vi "Runtime_Check.vi"(1 "Machine Settings":cluster{"Max Value":dbl, "Min Value":dbl}, 5 "Initial Timestamp":timestamp, 6 "error in (no error)":errorcluster, 7 "Tolerance":dbl, 8 "setpoint profile":cluster{"time (s)":dbl, "setpoint":dbl}[](array[cluster]), 9 "Process_REF":string) -> (0 "error out":errorcluster, 3 "Path Out":path)   [LabVIEW 2018]
panel:
  in  "stop":bool
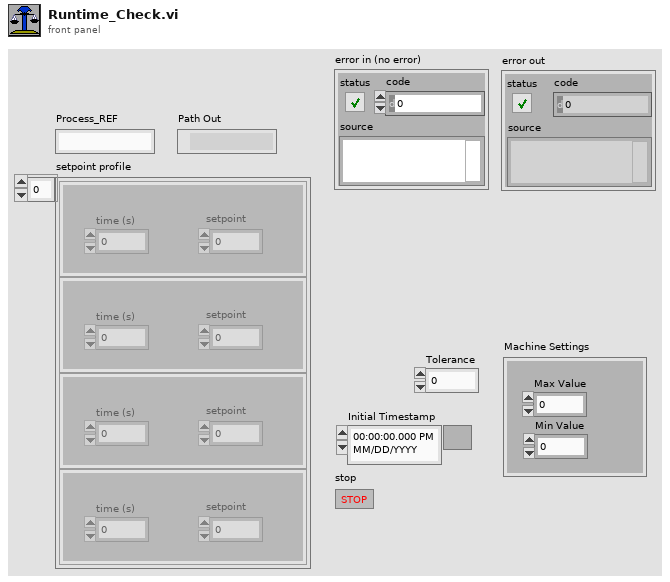
[diagram p1: front panel]
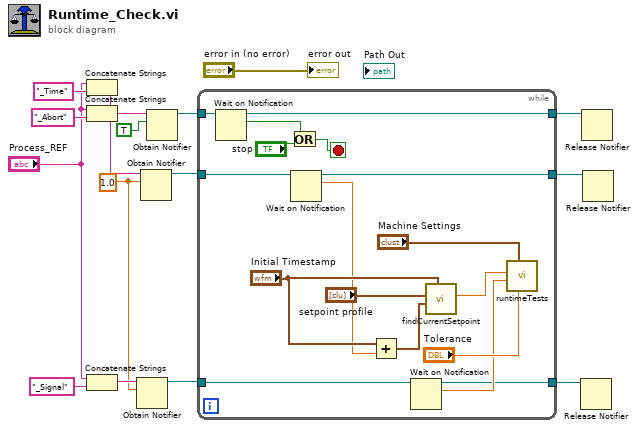
[diagram p0: block diagram]
diagram:
  w8 = 1.0
  n1 = Concatenate Strings("Process_REF", "_Time") -> (w11:string)
  n2 = Concatenate Strings("Process_REF", "_Abort") -> (w7:string)
  n3 = Concatenate Strings("Process_REF", "_Signal") -> (w10:string)
  n4 = Obtain Notifier(name (unnamed)=w10, notification data type=w8) -> (notifier out=w9:refnum<notifier>)  [unwired: 2 in, 2 out]
  n5 = Obtain Notifier(name (unnamed)=w11, notification data type=w8) -> (notifier out=w4:refnum<notifier>)  [unwired: 2 in, 2 out]
  n6 = Obtain Notifier(name (unnamed)=w7, notification data type=TRUE) -> (notifier out=w5:refnum<notifier>)  [unwired: 2 in, 2 out]
  n7 = while {
    tunnel: w4 -> [w22]
    tunnel: w9 -> [w23]
    tunnel: w5 -> [w19]
    tunnel: [w18] -> w3
    tunnel: [w21] -> w2
    tunnel: [w24] -> w1
    stop <- w26 stop-if-true
    n8 = Wait on Notification(notifier=w19) -> (notifier out=w18:refnum<notifier>, notification=w17:bool)  [unwired: 3 in, 2 out]
    n9 = Or(x=w17, y="stop") -> (x .or. y?=w26:bool)
    n10 = Wait on Notification(notifier=w22) -> (notifier out=w21:refnum<notifier>, notification=w20:dbl)  [unwired: 3 in, 2 out]
    n11 = Add(x="Initial Timestamp", y=w20) -> (x+y=w29:timestamp)
    n12 = Wait on Notification(notifier=w23) -> (notifier out=w24:refnum<notifier>, notification=w25:dbl)  [unwired: 3 in, 2 out]
    n13 = call "findCurrentSetpoint.vi"("Initial Timestamp"="Initial Timestamp", "Current Timestamp"=w29, "Setpoint Profile"="setpoint profile") -> ("Setpoint"=w32:dbl)  [unwired: 8 in]
    n14 = call "runtimeTests.vi"("Tolerance"="Tolerance", "Machine Settings"="Machine Settings", "Signal"=w25, "Setpoint"=w32) -> ()  [unwired: 7 in, 1 out]
  }
  n15 = Release Notifier(notifier=w1) -> ()  [unwired: 2 in, 3 out]
  n16 = Release Notifier(notifier=w3) -> ()  [unwired: 2 in, 3 out]
  n17 = Release Notifier(notifier=w2) -> ()  [unwired: 2 in, 3 out]
  "error out" <- "error in (no error)"
